vi "ABB Attendance report.vi"(10 "Report in":string) -> (2 "Report out":string)   [LabVIEW 2017]
uses:
  ABB global.vi
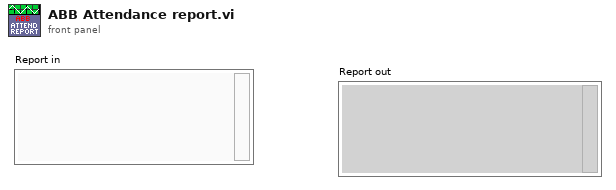
[diagram p1: front panel]
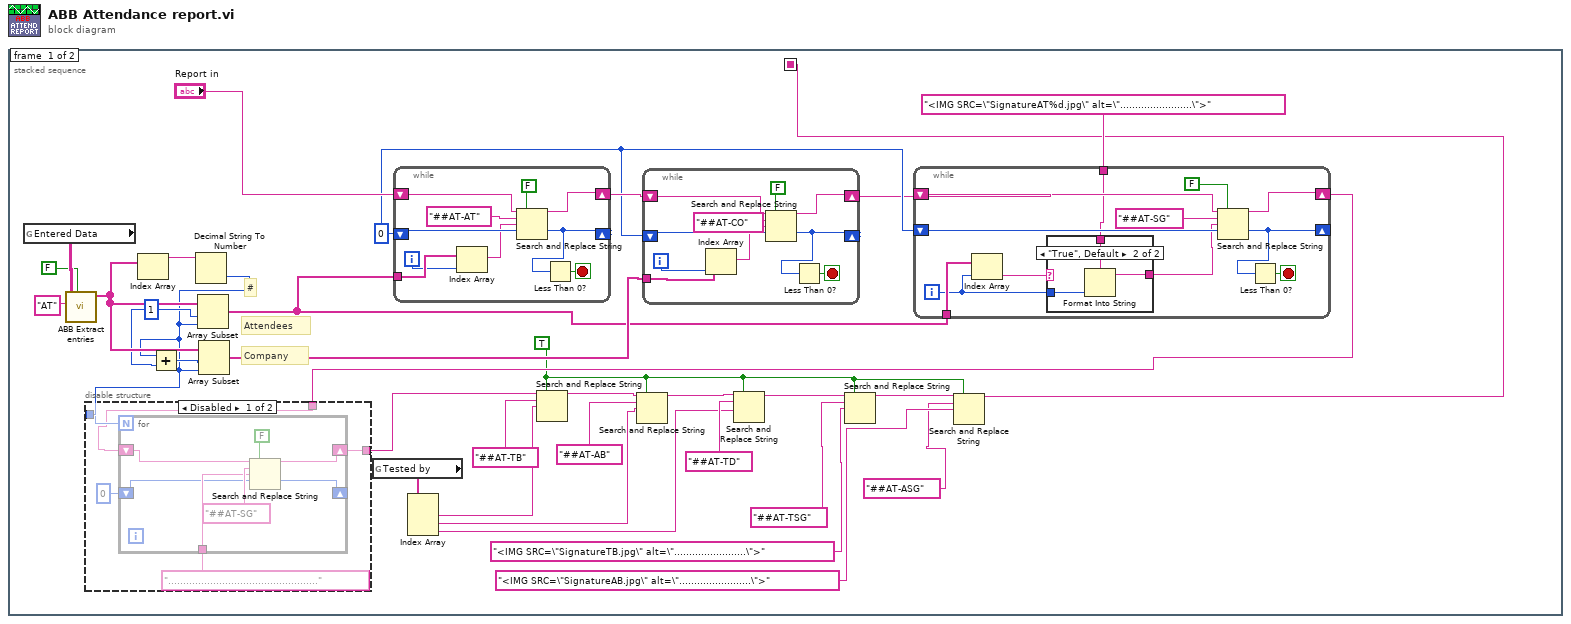
[diagram p0: block diagram]
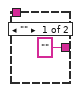
[diagram p3: hidden frame]
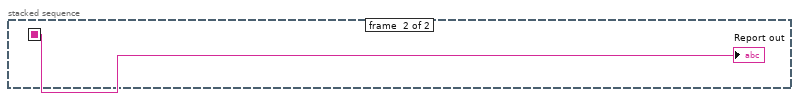
[diagram p4: hidden frame]
diagram:
  n1 = stacked-sequence {
    seq-local: [w4 _] -> [_ w84]
    frame #0 {
      w3 = TRUE ("replace all? (F)")
      w14 = 0
      w29 = 1 ("index")
      # "Company"
      # "Attendees"
      # "#"
      n2 = global read "ABB global.vi" "Entered Data"() -> (w31:string[][])
      n3 = call "ABB Extract entries.vi"("Pulldown text"=FALSE, "Entry ID"="AT", "Entry table in"=w31) -> ("Selected Entries"=w30:string[])  [unwired: 8 in]
      n4 = Index Array(array=w30) -> (element=w33:string)  [unwired: 1 in]
      n5 = Decimal String To Number(string=w33) -> (number=w16:i32)  [unwired: 2 in, 1 out]
      n6 = Add(x=w16, y=w29) -> (x+y=w28:i32)
      n7 = Array Subset(array=w30, index=w29, length=w16) -> (w10:string[])
      n8 = Array Subset(array=w30, index=w28, length=w16) -> (w26:string[])
      n9 = global read "ABB global.vi" "Tested by"() -> (w20:string[])
      n10 = while {
        shift-right: [w81] -> w27
        shift-left: "Report in" -> [w83]
        tunnel: w10 -> [w76]
        shift-right: [w77] -> _
        shift-left: w14 -> [w80]
        i -> [w75]
        stop <- w78 stop-if-true
        n11 = Index Array(array=w76, index=w75) -> (element=w74:string)
        n12 = Search and Replace String(replace all?=FALSE ("replace all? (F)"), input string=w83, search string="##AT-AT", replace string=w74, offset=w80) -> (result string=w81:string, offset past replacement=w77:i32)  [unwired: 3 in, 2 out]
        n13 = Less Than 0?(x=w77) -> (x < 0?=w78:bool)
      }
      n14 = Index Array(array=w20) -> (element #1=w19:string, element #2=w18:string, element #3=w17:string)  [unwired: 3 in]
      n15 = while {
        shift-right: [w71] -> w12
        shift-left: w27 -> [w73]
        tunnel: w26 -> [w66]
        shift-right: [w67] -> _
        shift-left: w14 -> [w70]
        i -> [w65]
        stop <- w68 stop-if-true
        n16 = Index Array(array=w66, index=w65) -> (element=w64:string)
        n17 = Search and Replace String(replace all?=FALSE ("replace all? (F)"), input string=w73, search string="##AT-CO", replace string=w64, offset=w70) -> (result string=w71:string, offset past replacement=w67:i32)  [unwired: 3 in, 2 out]
        n18 = Less Than 0?(x=w67) -> (x < 0?=w68:bool)
      }
      n19 = while {
        shift-right: [w57] -> w11
        shift-left: w12 -> [w59]
        shift-right: [w53] -> _
        shift-left: w14 -> [w56]
        tunnel: "<IMG SRC=\"SignatureAT%d.jpg\" alt=\"........................\">" -> [w51]
        tunnel: w10 -> [w50]
        i -> [w49]
        stop <- w54 stop-if-true
        n20 = Index Array(array=w50, index=w49) -> (element=w48:string)
        n21 = case shown="\"True\", Default" w48 {
          tunnel: ["" w63] -> w52
          tunnel: w51 -> [_ w62]
          tunnel: w49 -> [_ w61]
          frame "" {
          }
          frame "True", Default {
            n22 = Format Into String(format string=w62, w61) -> (resulting string=w63:string)  [unwired: 2 in, 1 out]
          }
        }
        n23 = Search and Replace String(replace all?=FALSE ("replace all? (F)"), input string=w59, search string="##AT-SG", replace string=w52, offset=w56) -> (result string=w57:string, offset past replacement=w53:i32)  [unwired: 3 in, 2 out]
        n24 = Less Than 0?(x=w53) -> (x < 0?=w54:bool)
      }
      n25 = disable-structure shown="Disabled" {
        disable-tunnel: w16 -> [w39 _]
        disable-tunnel: [w37 w47] -> w15
        disable-tunnel: w11 -> [w35 w47]
        frame Disabled {
          n26 = for {
            N: w39 -> [_]
            shift-right: [w42] -> w37
            shift-left: w35 -> [w43]
            tunnel: ".................................................." -> [w44]
            shift-right: [w40] -> _
            shift-left: 0 ("offset past replacement") -> [w41]
            n27 = Search and Replace String(replace all?=FALSE ("replace all? (F)"), input string=w43, search string="##AT-SG", replace string=w44, offset=w41) -> (result string=w42:string, offset past replacement=w40:i32)  [unwired: 3 in, 2 out]
          }
        }
        frame Enabled {
        }
      }
      n28 = Search and Replace String(replace all?=w3, input string=w15, search string="##AT-TB", replace string=w19) -> (result string=w25:string)  [unwired: 4 in, 3 out]
      n29 = Search and Replace String(replace all?=w3, input string=w25, search string="##AT-AB", replace string=w18) -> (result string=w24:string)  [unwired: 4 in, 3 out]
      n30 = Search and Replace String(replace all?=w3, input string=w24, search string="##AT-TD", replace string=w17) -> (result string=w9:string)  [unwired: 4 in, 3 out]
      n31 = Search and Replace String(replace all?=w3, input string=w9, search string="##AT-TSG", replace string="<IMG SRC=\"SignatureTB.jpg\" alt=\"........................\">") -> (result string=w6:string)  [unwired: 4 in, 3 out]
      n32 = Search and Replace String(replace all?=w3, input string=w6, search string="##AT-ASG", replace string="<IMG SRC=\"SignatureAB.jpg\" alt=\"........................\">") -> (result string=w4:string)  [unwired: 4 in, 3 out]
    }
    frame #1 {
      "Report out" <- w84
    }
  }
